vi "DeferFP.vi"(8 "error in":errorcluster, 11 "Defer Front Panel?":bool) -> (0 "error out":errorcluster)   [LabVIEW 2019, in "STS_LTRV.lvlib"]
uses:
  STS_LTRV.lvlib
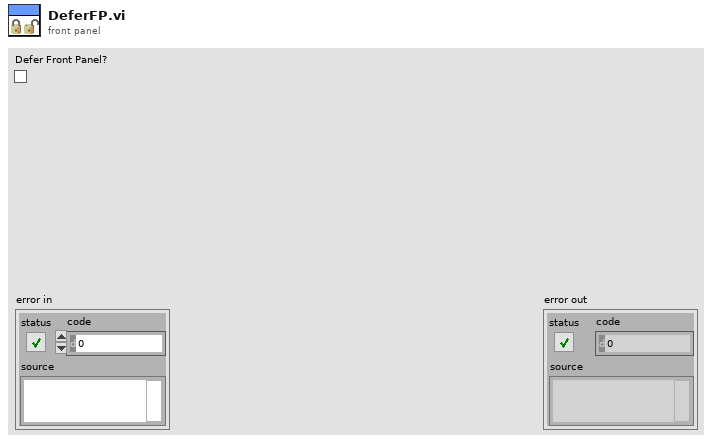
[diagram p1: front panel]
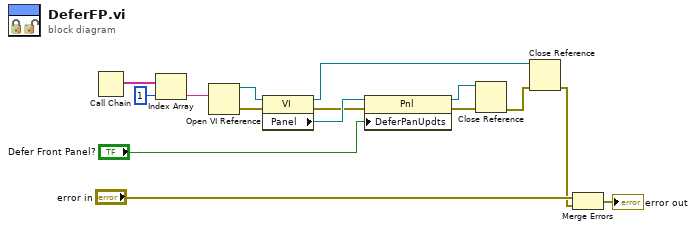
[diagram p0: block diagram]
diagram:
  n1 = Call Chain() -> (call chain=w15:string[])
  n2 = Index Array(array=w15, index=1) -> (element=w13:string)
  n3 = Open VI Reference(vi path=w13) -> (vi reference=w11:refnum<vi>, error out=w12:errorcluster)  [unwired: 5 in]
  n4 = property class="VI"(reference=w11, error in=w12) -> (reference out=w4:refnum<vi>, error out=w9:errorcluster, "Panel"=w10:refnum<vi>)
  n5 = property class="Pnl"(reference=w10, error in=w9, "DeferPanUpdts"="Defer Front Panel?") -> (reference out=w6:refnum<vi>, error out=w7:errorcluster)
  n6 = Close Reference(reference=w6, error in (no error)=w7) -> (error out=w5:errorcluster)
  n7 = Close Reference(reference=w4, error in (no error)=w5) -> (error out=w1:errorcluster)
  n8 = Merge Errors("error in", w1) -> (→"error out":errorcluster)
